vi "master.vi"() -> ()   [LabVIEW 2014]
uses:
  <vilib>/Instr/_visa.llb/VISA Configure Serial Port (Instr).vi
panel:
  in  "等待时间（毫秒）":u32
  out "电压2":dbl(graph)
  out "电压1":dbl(graph)
  out "转速表":dbl(graph)
  out "电压2":dbl
  out "电压1":dbl
  out "转速":dbl
  out "功能号返回":u32
  out "设备号返回":u32
  out "读取缓冲区":string
  out "发送帧":string
  in  "数据2":u16
  in  "数据1":u16
  in  "功能号":u8
  in  "设备号":u8
  in  "baud rate (9600)":u32=9600 caption="波特率(9600)"
  in  "VISA resource name":refnum<visa-resource-name> caption="VISA资源名称"
  in  "停止":bool
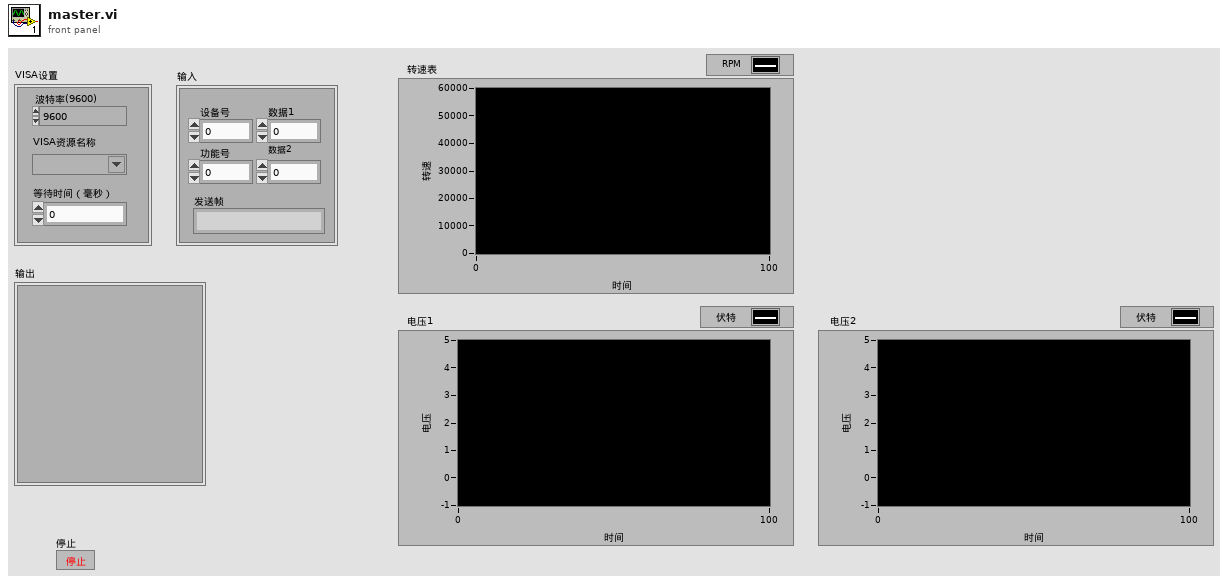
[diagram p1: front panel]
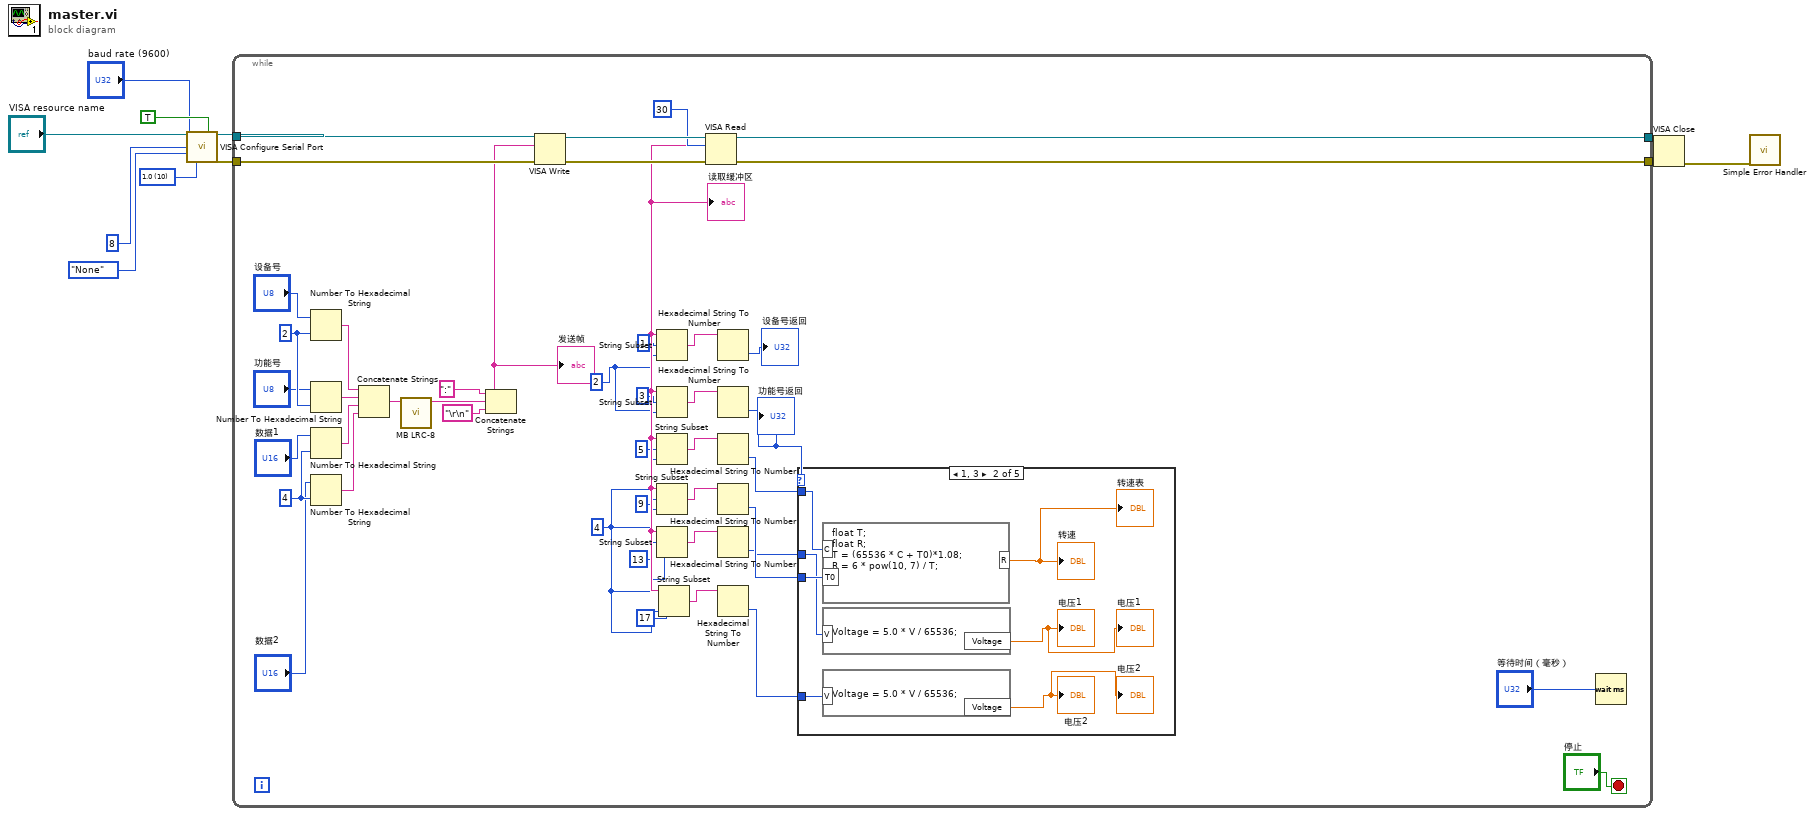
[diagram p0: block diagram]
diagram:
  w7 = u16 10 items=["1.0"=10, "1.5"=15, "2.0"=20] ("stop bits (10: 1 bit)")
  n1 = call-poly "VISA Configure Serial Port"("VISA resource name"="VISA resource name", "Enable Termination\nChar (T)"=TRUE ("Enable Termination\nChar (T)"), "baud rate (9600)"="baud rate (9600)", "data bits (8)"=u16 8, "parity (0:none)"=enum16{"None", "Odd", "Even", "Mark", "Space"}."None", "stop bits (10: 1 bit)"=w7) -> ("VISA resource name out"=w6:refnum<visa-resource-name>, "error out"=w5:errorcluster)  [unwired: 8 in]
  n2 = while {
    tunnel: w6 -> [w12]
    tunnel: w5 -> [w55]
    tunnel: [w53] -> w4
    tunnel: [w51] -> w3
    stop <- "停止" stop-if-true
    w25 = 4
    w26 = 2
    w49 = i16 2 ("宽度(-)")
    w48 = i16 4 ("宽度(-)")
    n3 = Number To Hexadecimal String(1:w49, 2:"设备号") -> (0:w43:string)
    n4 = Number To Hexadecimal String(1:w49, 2:"功能号") -> (0:w42:string)
    n5 = Number To Hexadecimal String(1:w48, 2:"数据1") -> (0:w41:string)
    n6 = Number To Hexadecimal String(1:w48, 2:"数据2") -> (0:w40:string)
    n7 = Concatenate Strings(w43, w42, w41, w40) -> (w36:string)
    n8 = call "MB LRC-8.vi"("String"=w36) -> ("string & LRC-8"=w38:string)  [unwired: 10 out]
    n9 = Concatenate Strings(":", w38, "\r\n") -> (w35:string)
    "发送帧" <- w35
    n10 = VISA Write(VISA resource name=w12, write buffer=w35, error in (no error)=w55) -> (VISA resource name out=w54:refnum<visa-resource-name>, error out=w52:errorcluster)  [unwired: 1 out]
    n11 = VISA Read(VISA resource name=w54, byte count=u32 30 ("字节总数"), error in (no error)=w52) -> (VISA resource name out=w53:refnum<visa-resource-name>, read buffer=w33:string, error out=w51:errorcluster)  [unwired: 1 out]
    "读取缓冲区" <- w33
    n12 = String Subset(string=w33, offset (0)=1 ("偏移量(0)"), length (rest)=w26) -> (substring=w18:string)
    n13 = String Subset(string=w33, offset (0)=3 ("偏移量(0)"), length (rest)=w26) -> (substring=w17:string)
    n14 = String Subset(string=w33, offset (0)=5 ("偏移量(0)"), length (rest)=w25) -> (substring=w16:string)
    n15 = String Subset(string=w33, offset (0)=9 ("偏移量(0)"), length (rest)=w25) -> (substring=w15:string)
    n16 = String Subset(string=w33, offset (0)=13 ("偏移量(0)"), length (rest)=w25) -> (substring=w14:string)
    n17 = String Subset(string=w33, offset (0)=17, length (rest)=w25) -> (substring=w13:string)
    n18 = Hexadecimal String To Number(string=w18) -> (number=→"设备号返回":u32)  [unwired: 1 in, 2 out]
    n19 = Hexadecimal String To Number(string=w17) -> (number=w23:u32)  [unwired: 1 in, 2 out]
    "功能号返回" <- w23
    n20 = Hexadecimal String To Number(string=w16) -> (number=w22:u32)  [unwired: 1 in, 2 out]
    n21 = Hexadecimal String To Number(string=w15) -> (number=w21:u32)  [unwired: 1 in, 2 out]
    n22 = Hexadecimal String To Number(string=w14) -> (number=w20:u32)  [unwired: 1 in, 2 out]
    n23 = Hexadecimal String To Number(string=w13) -> (number=w19:u32)  [unwired: 1 in, 2 out]
    n24 = case shown="1, 3" w23 {
      tunnel: w22 -> [_ w61 _ _ _]
      tunnel: w21 -> [_ w60 _ _ _]
      tunnel: w20 -> [_ w59 _ _ _]
      tunnel: w19 -> [_ w58 _ _ _]
      frame 0, Default {
      }
      frame 1, 3 {
        n25 = formula code="float T;\nfloat R;\nT = (65536 * C + T0)*1.08;\nR = 6 * pow(10, 7) / T;"("C"=w61, "T0"=w60) -> ("R"=→"转速" →"转速表":dbl)
        n26 = formula code="Voltage = 5.0 * V / 65536;"("V"=w59) -> ("Voltage"=→"电压1" →"电压1":dbl)
        n27 = formula code="Voltage = 5.0 * V / 65536;"("V"=w58) -> ("Voltage"=→"电压2" →"电压2":dbl)
      }
      frame 5 {
      }
      frame 4 {
      }
      frame 2 {
      }
    }
    n28 = Wait (ms)(milliseconds to wait="等待时间（毫秒）") -> ()  [unwired: 1 out]
  }
  n29 = VISA Close(VISA resource name=w4, error in (no error)=w3) -> (error out=w1:errorcluster)
  n30 = call <vilib>:"Simple Error Handler.vi"("error in (no error)"=w1) -> ()  [unwired: 4 in, 5 out]
